vi "Fitting test.vi"(0 "Input Array":dbl[](array[numeric]), 5 "Nb Pixel":dbl, 11 "error in (no error)":errorcluster) -> (4 "Best fit parameters":dbl[](array[numeric]), 6 "Residue":dbl format="%#_13g", 8 "Best fit":dbl[](array[numeric]), 14 "Covariance":dbl[][](array[numeric]), 15 "error out":errorcluster)   [LabVIEW 2014]
uses:
  <vilib>/gmath/NI_Gmath.lvlib
  <vilib>/gmath/NumericalOptimization/Nonlinear Curve Fit LM formula string.vi
  <vilib>/Analysis/NI_AALPro.lvlib
panel:
  out "Best nonlinear fit":dbl[](array[numeric])
  out "Waveform":waveform(dbl)
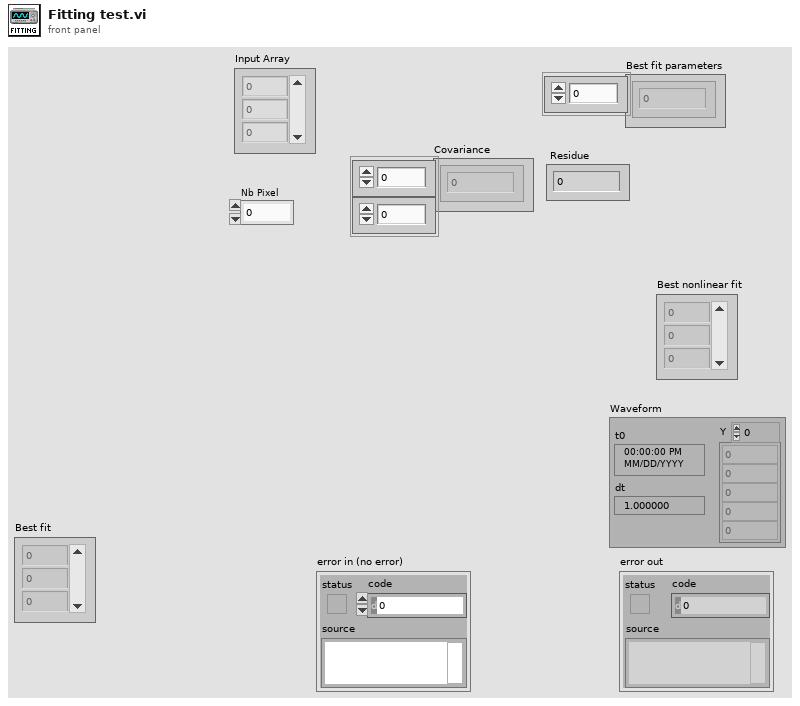
[diagram p1: front panel]
types:
  T1 = cluster{"model":string, "Parameters":string[], "x":string}
  T2 = typedef "NI_Matrix.lvlib/RealMatrix.ctl" = dbl[][]
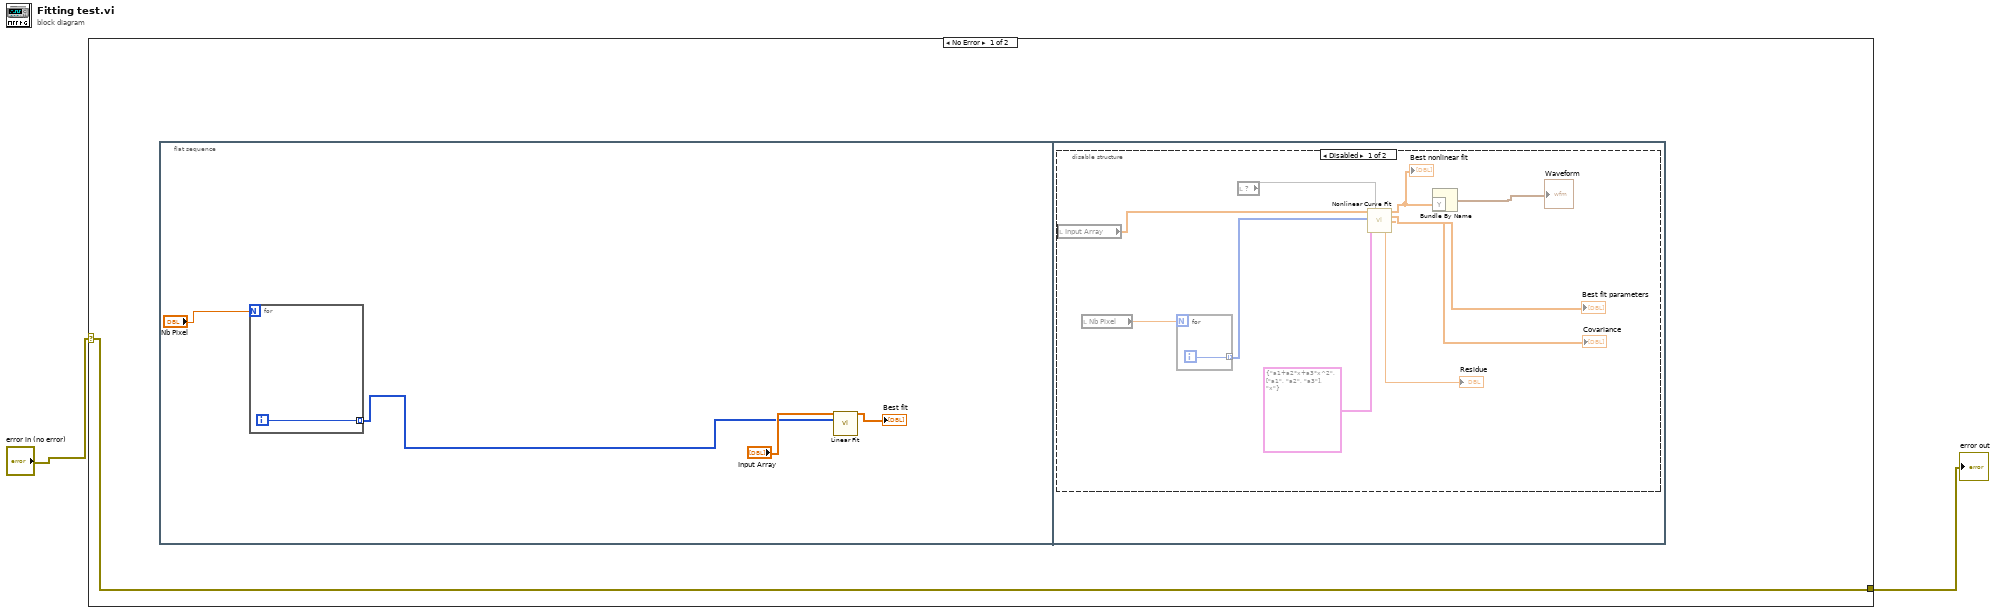
[diagram p0: block diagram]
diagram:
  n1 = case shown="No Error" "error in (no error)" {
    selector: "error in (no error)" -> [w3 w20]
    tunnel: [w3 w20] -> w1
    frame No Error {
      n2 = flat-sequence {
        frame #0 {
          n3 = for {
            N: "Nb Pixel" -> [_]
            tunnel: [w8] -> w5 mode=indexing
            i -> [w8]
          }
          n4 = call <vilib>:"Linear Fit.vi"("Y"="Input Array", "X"=w5) -> ("Best Linear Fit"=→"Best fit":dbl[])  [unwired: 9 in, 4 out]
        }
        frame #1 {
          n5 = disable-structure shown="Disabled" {
            frame Disabled {
              n6 = local read "Input Array"() -> (w17:dbl[])
              n7 = local read "Nb Pixel"() -> (w18:dbl)
              n8 = for {
                N: w18 -> [_]
                tunnel: [w19] -> w14 mode=indexing
                i -> [w19]
              }
              n9 = local read item#-1() -> (w9)
              n10 = call-poly <vilib>:"Nonlinear Curve Fit.vi"("Y"=w17, "initial parameters"=w9, "X"=w14, "model description"=T1 {"model"="a1+a2*x+a3*x^2", "Parameters"=["a1", "a2", "a3"], "x"="x"}) -> ("best nonlinear fit"=w16:dbl[], "best fit parameters"=→"Best fit parameters":dbl[], "covariance"=→"Covariance":T2, "residue"=→"Residue":dbl)  [unwired: 7 in, 1 out]
              "Best nonlinear fit" <- w16
              n11 = Bundle By Name("Y"=w16) -> (→"Waveform":waveform(dbl))  [unwired: 1 in]
            }
            frame Enabled {
            }
          }
        }
      }
    }
    frame Error {
    }
  }
  "error out" <- w1
